vi "Coder.vi"(1 "Station Address":u32, 7 "Input":string) -> (8 "Output":string)   [LabVIEW 2010, in "DCP551.lvlib"]
uses:
  DCP551.lvlib
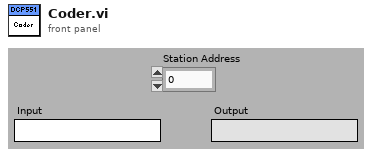
[diagram p1: front panel]
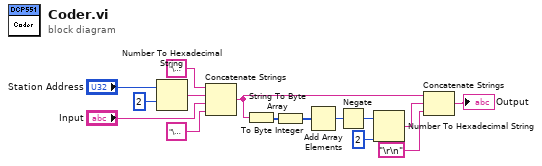
[diagram p0: block diagram]
diagram:
  n1 = Number To Hexadecimal String(1:i16 2 ("width (-)"), 2:"Station Address") -> (0:w7:string)
  n2 = Concatenate Strings("\u0002" ("string"), w7, "Input", "\u0003" ("string")) -> (w2:string)
  n3 = String To Byte Array(string=w2) -> (unsigned byte array=w13:u8[])
  n4 = To Byte Integer(number=w13) -> (8bit integer=w14:i8[])
  n5 = Add Array Elements(numeric array=w14) -> (sum=w11:i8)
  n6 = Negate(x=w11) -> (-x=w12:i8)
  n7 = Number To Hexadecimal String(1:i16 2 ("width (-)"), 2:w12) -> (0:w10:string)
  n8 = Concatenate Strings(w2, w10, "\r\n") -> (→"Output":string)
